vi "Find Function from Notifier Name.vi"(7 "Unique Notifier Name":string) -> (8 "Function":T1)   [LabVIEW 2020]
uses:
  Hardware Configuration Controls/Device Function.ctl
panel:
  in  "Device Function":T1=enum."405 nm Excitation"
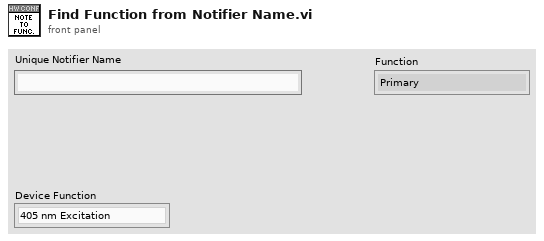
[diagram p1: front panel]
types:
  T1 = typedef "Device Function.ctl" = enum16{"Primary", "Secondary", "Overview", "Wide Field Drift Correction", "642 nm Excitation", "560 nm Excitation", "940 nm Excitation", "546 nm Excitation", "488 nm Excitation", "405 nm Excitation", "Objective Drift Correction", "4Pi Objective Lock", "Objective XY", "Objective Z", "Sample XY", "Sample Coarse Z", "Sample Z", "4Pi Lower", "4Pi Upper", "Mojo", "Adj Cavity", "Line Scanning", "Alert"}
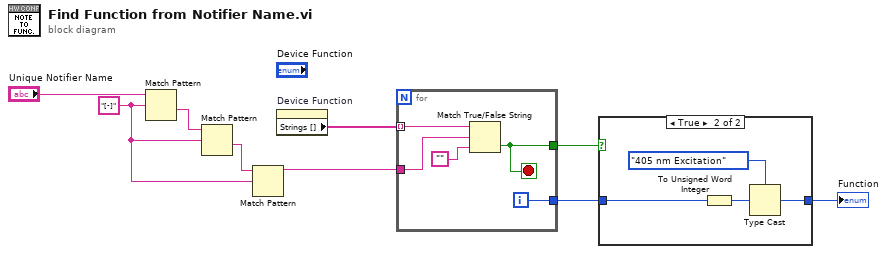
[diagram p0: block diagram]
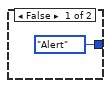
[diagram p2: hidden frame]
diagram:
  w7 = "[-]" ("regular expression")
  n1 = Match Pattern(string="Unique Notifier Name", regular expression=w7) -> (after substring=w9:string)  [unwired: 1 in, 3 out]
  n2 = Match Pattern(string=w9, regular expression=w7) -> (after substring=w8:string)  [unwired: 1 in, 3 out]
  n3 = Match Pattern(string=w8, regular expression=w7) -> (before substring=w6:string)  [unwired: 1 in, 3 out]
  n4 = property on="Device Function" class="Enum (strict)"() -> ("Strings []"=w5:string[])  [unwired: 2 in, 2 out]
  n5 = for {
    tunnel: w6 -> [w13]
    tunnel: w5 -> [w14] mode=indexing
    tunnel: [w12] -> w4
    tunnel: [w11] -> w2
    i -> [w12]
    stop <- w11 stop-if-true
    n6 = Match True/False String(2:"", 3:w13, 4:w14) -> (0:w11:bool)  [unwired: 1 out]
  }
  n7 = case shown="True" w2 {
    tunnel: w4 -> [_ w17]
    tunnel: [Device_Function."Alert" ("Device Function") w16] -> w3
    frame False {
    }
    frame True {
      n8 = To Unsigned Word Integer(number=w17) -> (unsigned 16bit integer=w18:u16)
      n9 = Type Cast(type=Device_Function."405 nm Excitation" ("Device Function"), x=w18) -> (*(type *) &x=w16:T1)
    }
  }
  "Function" <- w3
